vi "Insert Start Message.vi"(8 "error in (no error)":errorcluster, 10 "Start Time":timestamp, 11 "AcquireTraces in":refnum<class "AcquireTraces.lvclass">) -> (0 "error out":errorcluster, 3 "AcquireTraces out":refnum<class "AcquireTraces.lvclass">)   [LabVIEW 2014, in "AcquireTraces.lvclass"]
uses:
  AcquireTraces.lvclass
  AcquistionObject/AcquistionObject.lvclass
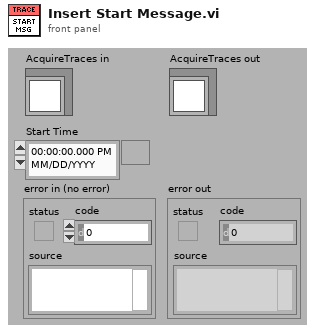
[diagram p1: front panel]
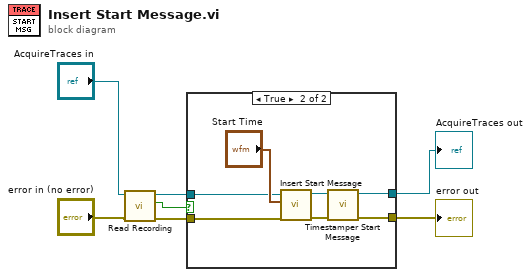
[diagram p0: block diagram]
diagram:
  n1 = call-dynamic "Read Recording.vi"("error in (no error)"="error in (no error)", "AcquireTraces in"="AcquireTraces in") -> ("error out"=w4:errorcluster, "Recording"=w1:bool, "AcquireTraces out"=w2:refnum<class "AcquireTraces.lvclass">)  [unwired: 7 in]
  n2 = case shown="True" w1 {
    tunnel: [w8 w13] -> w7
    tunnel: [w9 w12] -> w6
    tunnel: w4 -> [w8 w11]
    tunnel: w2 -> [w9 w10]
    frame False {
    }
    frame True {
      n3 = call-parent "Insert Start Message.vi"("error in (no error)"=w11, "Start Time"="Start Time", "AcquistionObject in"=w10) -> ("error out"=w14:errorcluster, "AcquistionObject out"=w15:refnum<class "AcquireTraces.lvclass">)  [unwired: 7 in]
      n4 = call-dynamic "Timestamper Start Message.vi"("error in (no error)"=w14, "AcquistionObject in"=w15) -> ("error out"=w13:errorcluster, "AcquistionObject out"=w12:refnum<class "AcquireTraces.lvclass">)  [unwired: 8 in]
    }
  }
  "error out" <- w7
  "AcquireTraces out" <- w6
